vi "Create.vi"(7 "gRPC server ID":T1, 8 "error in":errorcluster, 9 "measurement service in":refnum<class "IMeasurement Service.lvclass">, 10 "measurement plugin service in":refnum<class "Measurement Plugin Service.lvclass">, 11 "pin map context":T2) -> (0 "error out":errorcluster, 3 "measure call context out":refnum<class "Measure Call Context.lvclass">)   [LabVIEW 2021, in "NI Measurement Plug-In SDK.lvlib" / "Measure Call Context.lvclass"]
uses:
  Measure Call Context.lvclass
  Helpers/TypeDefs/Pin Map Context.ctl
  <vilib>/gRPC/LabVIEW gRPC Library/Shared/grpcId.ctl
  IMeasurement Service/IMeasurement Service.lvclass
  Measurement Plugin Service/Measurement Plugin Service.lvclass
  Data.ctl
  gRPC/Generated APIs/ni/measurementlink/sessionmanagement/v1/RPC Messages/ni_measurementlink_sessionmanagement_v1_SessionInformation.ctl
  gRPC/Generated APIs/ni/measurementlink/sessionmanagement/v1/RPC Messages/nidevice_grpc_Session.ctl
  gRPC/Generated APIs/ni/measurementlink/sessionmanagement/v1/RPC Messages/ni_measurementlink_sessionmanagement_v1_ChannelMapping.ctl
  Measure Call Context.lvclass/Measure Call Context.ctl
  NI Measurement Plug-In SDK.lvlib
  <vilib>/gRPC/LabVIEW gRPC Library/grpc-lvsupport-release.lvlib
  gRPC/Generated APIs/ni/measurementlink/sessionmanagement/v1/ni.measurementlink.sessionmanagement.v1.api.lvlib
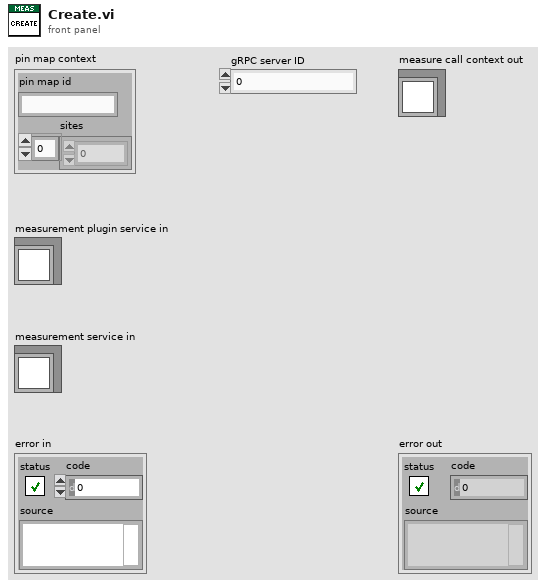
[diagram p1: front panel]
types:
  T1 = typedef "grpc-lvsupport-release.lvlib/grpcId.ctl" = u64
  T2 = typedef "NI Measurement Plug-In SDK.lvlib/Pin Map Context.ctl" = cluster{"pin map id":string, "sites":i32[]}
  T3 = typedef "NI Measurement Plug-In SDK.lvlib/Measure Call Context.lvclass/Data.ctl" = cluster{"pin map context":T2, "gRPC ID":T1, "measurement service":refnum<class "IMeasurement Service.lvclass">, "measurement plugin service":refnum<class "Measurement Plugin Service.lvclass">, "reserved session infos":set{T4}}
  T4 = typedef "ni.measurementlink.sessionmanagement.v1.api.lvlib/ni_measurementlink_sessionmanagement_v1_SessionInformation.ctl" = cluster{"session":T5, "resource_name":string, "channel_list":string, "instrument_type_id":string, "session_exists":bool, "channel_mappings":T6[]}
  T5 = typedef "ni.measurementlink.sessionmanagement.v1.api.lvlib/nidevice_grpc_Session.ctl" = cluster{"name":string}
  T6 = typedef "ni.measurementlink.sessionmanagement.v1.api.lvlib/ni_measurementlink_sessionmanagement_v1_ChannelMapping.ctl" = cluster{"pin_or_relay_name":string, "site":i32, "channel":string, "multiplexer_resource_name":string, "multiplexer_route":string}
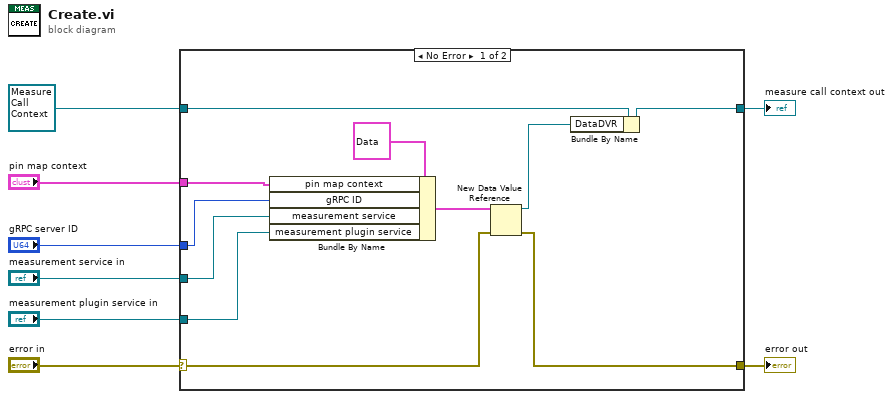
[diagram p0: block diagram]
diagram:
  n1 = case shown="No Error" "error in" {
    selector: "error in" -> [w12 w21]
    tunnel: [w9 w21] -> w7
    tunnel: [w18 w20] -> w6
    tunnel: refnum<class "Measure Call Context.lvclass"> refnum ("MeasurementContext.lvclass") -> [w19 w20]
    tunnel: "pin map context" -> [w16 _]
    tunnel: "gRPC server ID" -> [w15 _]
    tunnel: "measurement service in" -> [w14 _]
    tunnel: "measurement plugin service in" -> [w13 _]
    frame No Error {
      n2 = Bundle By Name(cluster=T3 {"pin map context"={"pin map id"="", "sites"=[]}, "gRPC ID"=0, "measurement service"=refnum, "measurement plugin service"=refnum, "reserved session infos"={}} ("Data"), "pin map context"=w16, "gRPC ID"=w15, "measurement service"=w14, "measurement plugin service"=w13) -> (w11:T3)
      n3 = New Data Value Reference(data value=w11, error in=w12) -> (data value reference=w10:refnum<data-value>, error out=w9:errorcluster)
      n4 = Bundle By Name(cluster=w19, "DataDVR"=w10) -> (w18:refnum<class "Measure Call Context.lvclass">)
    }
    frame Error {
    }
  }
  "error out" <- w7
  "measure call context out" <- w6
